vi "DO_init1.vi"(6 "conninfo":T1={"host"="localhost", "port"="5432", "client_encoding"="WIN1251", "dbname"="data", "user"="postgres", "password"=""}, 7 "N_param":i32, 9 "Names def":string[][](array[string]), 10 "Parameters def":dbl[][](array[numeric]), 11 "DO_fcode_full":string[](array[string])) -> (0 "error":errorcluster, 1 "DONames":refnum<data-value>, 2 "DOP":refnum<data-value>, 3 "DO_defs":T3)   [LabVIEW 2019]
uses:
  Inputs.lvlib
  Ctl/Parameter State.ctl
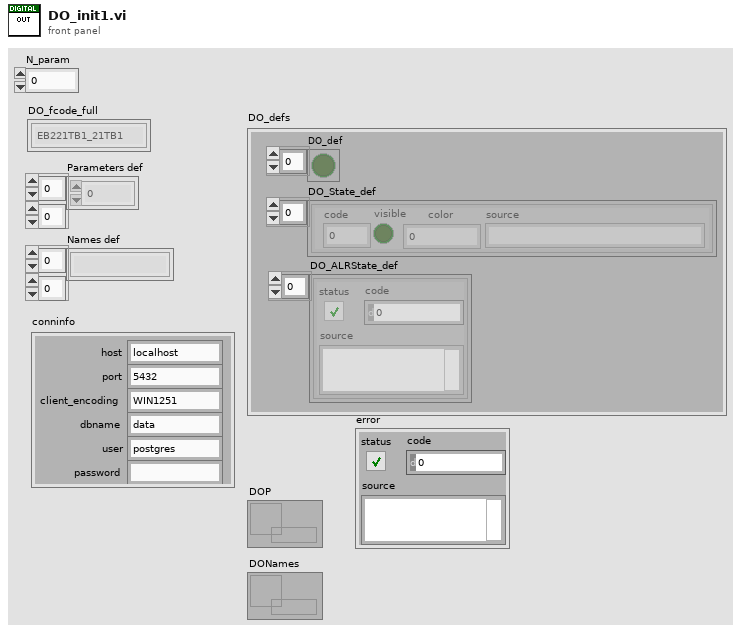
[diagram p1: front panel]
types:
  T1 = cluster{"host":string, "port":string, "client_encoding":string, "dbname":string, "user":string, "password":string}
  T2 = typedef "Inputs.lvlib/Parameter State.ctl" = cluster{"code":i32, "visible":bool, "color":u32, "source":string}
  T3 = cluster{"DO_def":bool[], "DO_State_def":T2[], "DO_ALRState_def":errorcluster[]}
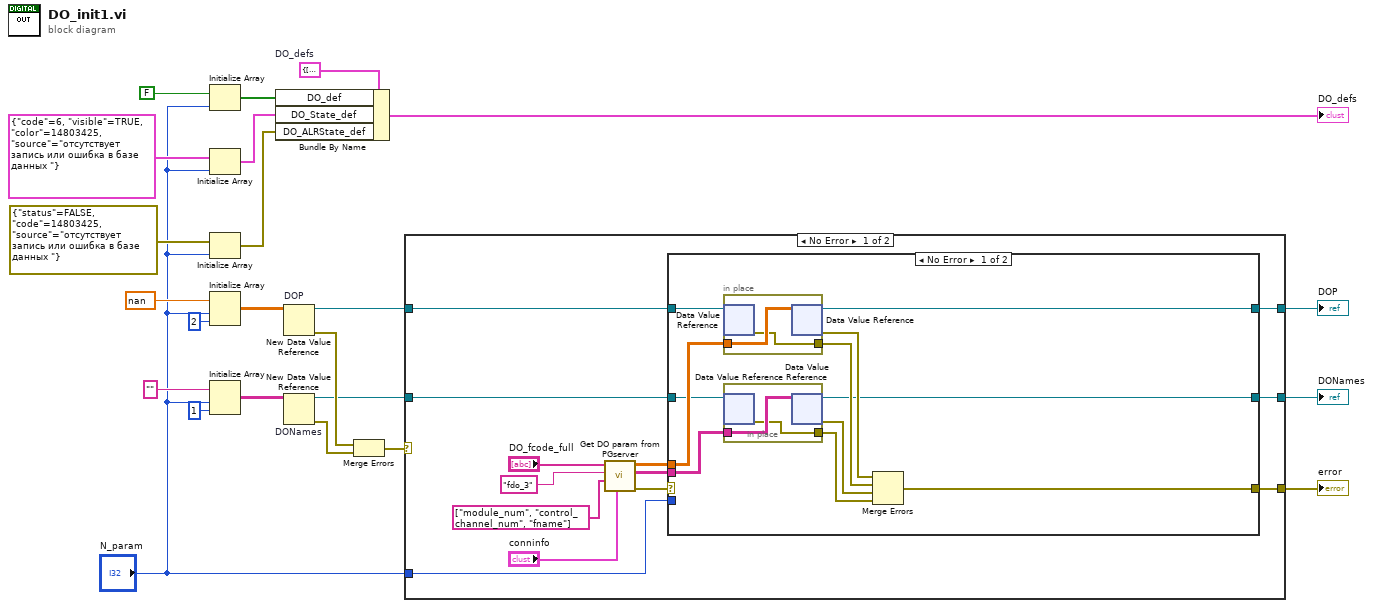
[diagram p0: block diagram]
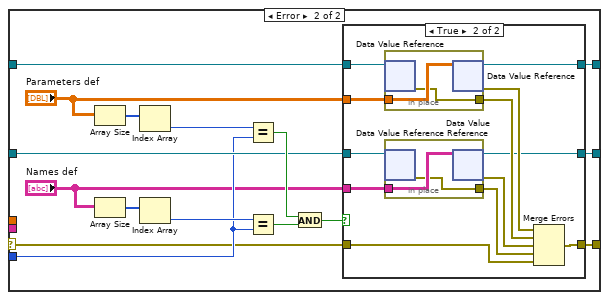
[diagram p2: hidden frame]
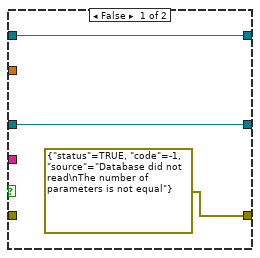
[diagram p3: hidden frame]
diagram:
  w10 = T3 {"DO_def"=[], "DO_State_def"=[], "DO_ALRState_def"=[]}  # DO_defs
  n1 = Initialize Array(FALSE, "N_param") -> (w22:bool[])
  n2 = Initialize Array(T2 {"code"=6, "visible"=TRUE, "color"=14803425, "source"="отсутствует запись или ошибка в базе данных "} ("STATE"), "N_param") -> (w21:T2[])
  n3 = Initialize Array(errorcluster {"status"=FALSE, "code"=14803425, "source"="отсутствует запись или ошибка в базе данных "} ("ALRSTATE"), "N_param") -> (w20:errorcluster[])
  n4 = Initialize Array(nan ("DIP"), "N_param", 2 ("dimension size")) -> (w14:dbl[][])
  n5 = Initialize Array("" ("DINames"), "N_param", 1 ("dimension size")) -> (w13:string[][])
  n6 = Bundle By Name(cluster=w10, "DO_def"=w22, "DO_State_def"=w21, "DO_ALRState_def"=w20) -> (→"DO_defs":T3)
  n7 = New Data Value Reference "DOP"(data value=w14) -> (data value reference=w7:refnum<data-value>, error out=w12:errorcluster)  [unwired: 1 in]
  n8 = New Data Value Reference "DONames"(data value=w13) -> (data value reference=w5:refnum<data-value>, error out=w11:errorcluster)  [unwired: 1 in]
  n9 = Merge Errors(w12, w11) -> (w4:errorcluster)
  n10 = case shown="No Error" w4 {
    selector: w4 -> [_ w89]
    tunnel: w7 -> [w36 w88]
    tunnel: w5 -> [w35 w87]
    tunnel: "N_param" -> [w31 _]
    tunnel: [w34 w89] -> w1
    tunnel: [w33 w88] -> w6
    tunnel: [w32 w87] -> w2
    frame No Error {
      n11 = call "Get DO param from PGserver.vi"("conninfo"="conninfo", "DOParamColumns"=string[] ["module_num", "control_channel_num", "fname"], "DOParamTable"="fdo_3" ("DIParamTable"), "DO_fcode_full"="DO_fcode_full") -> ("error out"=w25:errorcluster, "Names table"=w26:string[][], "DOParameters table"=w27:dbl[][])  [unwired: 5 in]
      n12 = case shown="No Error" w25 {
        selector: w25 -> [_ w55]
        tunnel: w27 -> [w46 _]
        tunnel: w26 -> [w44 _]
        tunnel: [w37 w56] -> w34
        tunnel: w36 -> [w47 w61]
        tunnel: w35 -> [w45 w60]
        tunnel: [w39 w58] -> w33
        tunnel: [w38 w57] -> w32
        tunnel: w31 -> [_ w59]
        frame No Error {
          n13 = in-place {
            in-place-border: w46 -> [w49]
            in-place-border: [w48] -> w42
            n14 = in-place-dvr #1(w47) -> (w48:errorcluster)  [unwired: 1 out]
            n15 = in-place-dvr #1(w49) -> (w39:refnum<data-value>, w43:errorcluster)
          }
          n16 = in-place {
            in-place-border: w44 -> [w51]
            in-place-border: [w50] -> w40
            n17 = in-place-dvr #2(w45) -> (w50:errorcluster)  [unwired: 1 out]
            n18 = in-place-dvr #2(w51) -> (w38:refnum<data-value>, w41:errorcluster)
          }
          n19 = Merge Errors(w43, w42, w41, w40) -> (w37:errorcluster)
        }
        frame Error {
          n20 = Array Size(array="Parameters def") -> (size(s)=w62:i32[])
          n21 = Array Size(array="Names def") -> (size(s)=w63:i32[])
          n22 = Index Array(array=w62) -> (element=w64:i32)  [unwired: 1 in]
          n23 = Index Array(array=w63) -> (element=w65:i32)  [unwired: 1 in]
          n24 = Equal?(x=w64, y=w59) -> (x = y?=w66:bool)
          n25 = Equal?(x=w65, y=w59) -> (x = y?=w67:bool)
          n26 = And(x=w66, y=w67) -> (x .and. y?=w54:bool)
          n27 = case shown="True" w54 {
            tunnel: "Parameters def" -> [_ w81]
            tunnel: "Names def" -> [_ w79]
            tunnel: [errorcluster {"status"=TRUE, "code"=-1, "source"="Database did not read\nThe number of parameters is not equal"} ("ALRSTATE") w72] -> w56
            tunnel: w61 -> [w70 w82]
            tunnel: w60 -> [w69 w80]
            tunnel: [w70 w74] -> w58
            tunnel: [w69 w73] -> w57
            tunnel: w55 -> [_ w71]
            frame False {
            }
            frame True {
              n28 = in-place {
                in-place-border: w81 -> [w84]
                in-place-border: [w83] -> w77
                n29 = in-place-dvr #3(w82) -> (w83:errorcluster)  [unwired: 1 out]
                n30 = in-place-dvr #3(w84) -> (w74:refnum<data-value>, w78:errorcluster)
              }
              n31 = in-place {
                in-place-border: w79 -> [w86]
                in-place-border: [w85] -> w75
                n32 = in-place-dvr #4(w80) -> (w85:errorcluster)  [unwired: 1 out]
                n33 = in-place-dvr #4(w86) -> (w73:refnum<data-value>, w76:errorcluster)
              }
              n34 = Merge Errors(w78, w77, w76, w75, w71) -> (w72:errorcluster)
            }
          }
        }
      }
    }
    frame Error {
    }
  }
  "error" <- w1
  "DOP" <- w6
  "DONames" <- w2
